vi "Autosort Add Sort Option.vi"(8 "error in (no error)":errorcluster, 11 "Autosort Parameters":T1) -> (0 "error out":errorcluster, 3 "Num Sets":i32)   [LabVIEW 2016]
uses:
  Autosort Parameters.ctl
  Autosort Parameters Set.vi
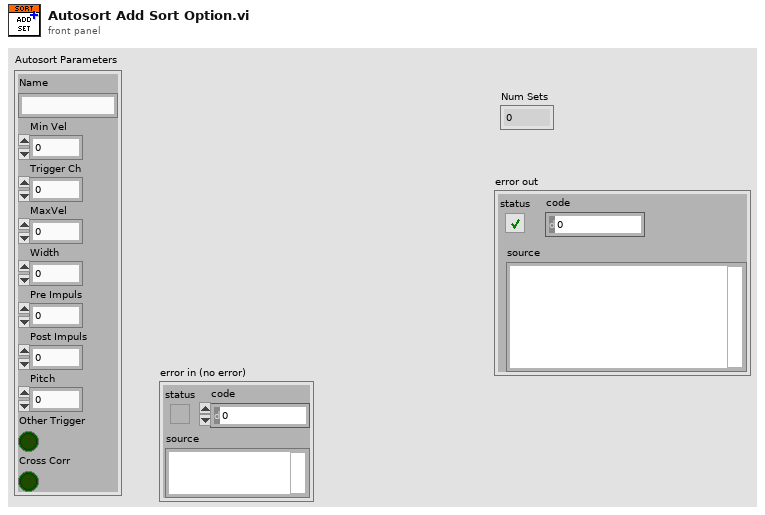
[diagram p1: front panel]
types:
  T1 = typedef "Autosort Parameters.ctl" = cluster{"Name":string, "Min Vel":dbl, "Trigger Ch":i32, "MaxVel":dbl, "Width":i32, "Pre Impuls":i32, "Post Impuls":i32, "Pitch":dbl, "Other Trigger":bool, "Cross Corr":bool}
  T2 = enum16{"open", "replace", "create", "open or create", "replace or create", "replace or create with confirmation"}
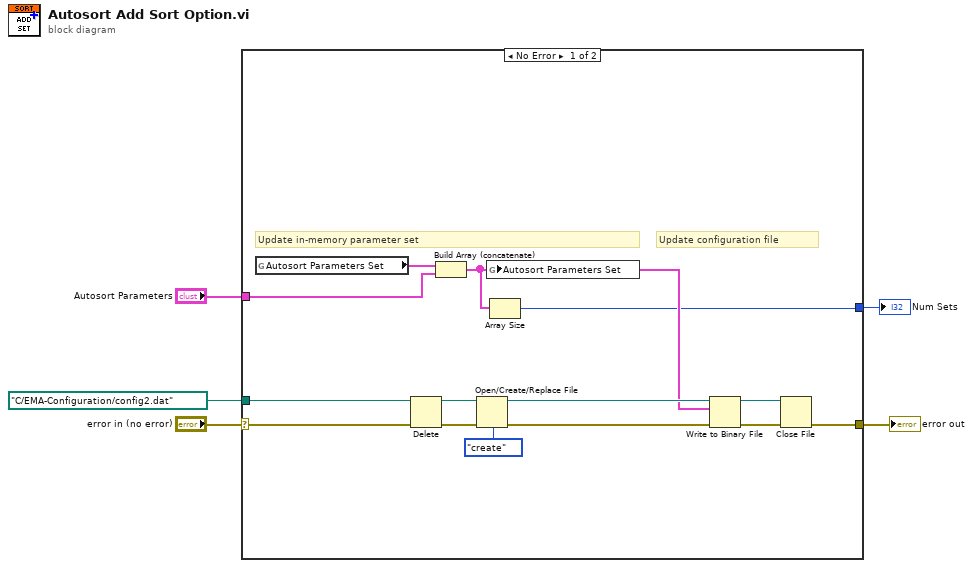
[diagram p0: block diagram]
diagram:
  n1 = case shown="No Error" "error in (no error)" {
    selector: "error in (no error)" -> [w16 w20]
    tunnel: "Autosort Parameters" -> [w19 _]
    tunnel: [w8 w20] -> w3
    tunnel: path "C:/EMA-Configuration/config2.dat" ("path") -> [w17 _]
    tunnel: [w6 _] -> w1
    frame No Error {
      # "Update configuration file"
      # "Update in-memory parameter set"
      n2 = global read "Autosort Parameters Set.vi" "Autosort Parameters Set"() -> (w18:T1[])
      n3 = Delete(path (use dialog)=w17, error in=w16) -> (deleted path=w15:path, error out=w14:errorcluster)  [unwired: 3 in, 1 out]
      n4 = Build Array (concatenate)(w18, w19) -> (w7:T1[])
      n5 = Open/Create/Replace File(file path (use dialog)=w15, error in=w14, operation (0:open)=T2."create") -> (refnum out=w12:refnum<file>, error out=w11:errorcluster)  [unwired: 3 in, 1 out]
      n6 = global write "Autosort Parameters Set.vi" "Autosort Parameters Set"(w7) -> ()
      n7 = Array Size(array=w7) -> (size(s)=w6:i32)
      n8 = Write to Binary File(file (use dialog)=w12, data=w7, error in=w11) -> (refnum out=w9:refnum<file>, error out=w10:errorcluster)  [unwired: 3 in, 1 out]
      n9 = Close File(refnum=w9, error in=w10) -> (error out=w8:errorcluster)  [unwired: 1 out]
    }
    frame Error {
    }
  }
  "error out" <- w3
  "Num Sets" <- w1
